vi "CAL-Update Value.vi"(0 "path":path, 5 "Frequency (kHz)":dbl, 7 "Ceiling (dB SPL)":dbl, 11 "error in (no error)":errorcluster) -> (15 "error out":errorcluster)   [LabVIEW 2020]
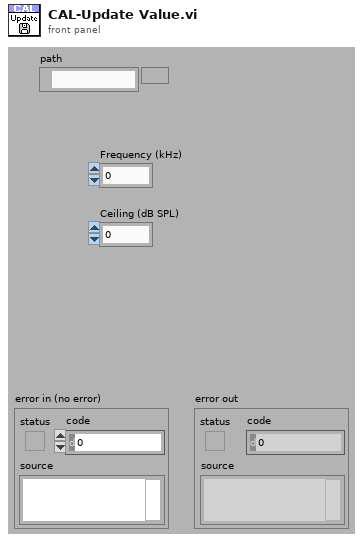
[diagram p1: front panel]
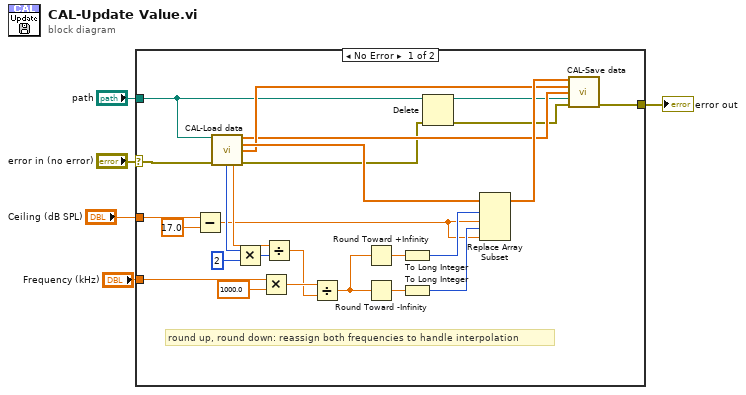
[diagram p0: block diagram]
diagram:
  n1 = case shown="No Error" "error in (no error)" {
    selector: "error in (no error)" -> [w31 w32]
    tunnel: [w12 w32] -> w5
    tunnel: "path" -> [w9 _]
    tunnel: "Frequency (kHz)" -> [w28 _]
    tunnel: "Ceiling (dB SPL)" -> [w18 _]
    frame No Error {
      # "round up, round down: reassign both frequencies to handle interpolation"
      n2 = Subtract(x=w18, y=17.0) -> (x-y=w16:dbl)
      n3 = call "CAL-Load data.vi"("user path"=w9, "error in (no error)"=w31) -> ("Frequency (Hz)"=w13:dbl[], "Mag"=w21:dbl[], "Phase"=w14:dbl[], "npts"=w29:i32, "Fs (Hz)"=w30:dbl, "error out"=w7:errorcluster)  [unwired: 6 in, 2 out]
      n4 = Multiply(x=w29, y=2) -> (x*y=w11:i32)
      n5 = Multiply(x=w28, y=1000.0) -> (x*y=w26:dbl)
      n6 = Divide(x=w30, y=w11) -> (x/y=w25:dbl)
      n7 = Divide(x=w26, y=w25) -> (x/y=w24:dbl)
      n8 = Round Toward +Infinity(x=w24) -> (ceil(x): smallest int >= x=w23:dbl)
      n9 = Round Toward -Infinity(1:w24) -> (0:w22:dbl)
      n10 = To Long Integer(number=w23) -> (32bit integer=w20:i32)
      n11 = To Long Integer(number=w22) -> (32bit integer=w19:i32)
      n12 = Delete(path (use dialog)=w9, error in=w7) -> (deleted path=w8:path, error out=w6:errorcluster)  [unwired: 3 in, 1 out]
      n13 = Replace Array Subset(array=w21, new element #1=w16, index #1=w20, new element #2=w16, index #2=w19) -> (w15:dbl[])
      n14 = call "CAL-Save data.vi"("Mag"=w15, "Phase"=w14, "Frequency"=w13, "path"=w8, "error in (no error)"=w6) -> ("error out"=w12:errorcluster)  [unwired: 9 in, 1 out]
    }
    frame Error {
    }
  }
  "error out" <- w5
